vi "DeQueue Ball Element.vi"() -> (3 "Ball Images":T1[](array[typedef]))   [LabVIEW 2019]
uses:
  <vilib>/vision/Image Controls.llb/IMAQ Image.ctl
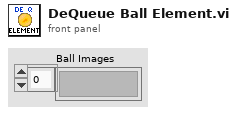
[diagram p1: front panel]
types:
  T1 = typedef "IMAQ Image.ctl" = refnum<image>
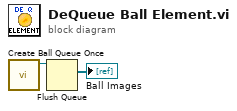
[diagram p0: block diagram]
diagram:
  n1 = call "Create Ball Queue Once.vi"() -> ("queue out"=w2:refnum<queue>)  [unwired: 11 in]
  n2 = Flush Queue(queue=w2) -> (remaining elements=→"Ball Images":T1[])  [unwired: 1 in, 2 out]
